vi "MQTT 3.1.1 Constant.vi"() -> (3 "MQTT 3.1.1":refnum<class "MQTTVersion.lvclass">)   [LabVIEW 2013, in "MQTT_Control_Packets.lvlib" / "MQTTVersion.lvclass"]
uses:
  MQTTVersion.lvclass
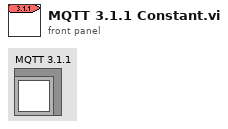
[diagram p1: front panel]
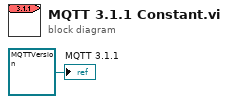
[diagram p0: block diagram]
diagram:
  "MQTT 3.1.1" <- refnum<class "MQTTVersion.lvclass"> refnum ("MQTT 3.1.1")
